vi "testZone.vi"() -> ()   [LabVIEW 2023]
uses:
  zones.ctl
  Zone.lvclass
  Field_class/Field.lvclass
panel:
  out "Zone":T1
  in  "Point":dbl[](array[numeric])
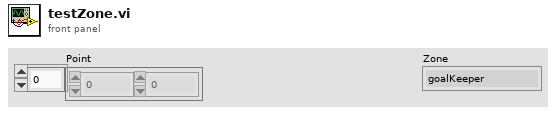
[diagram p1: front panel]
types:
  T1 = typedef "Zone.lvclass/zones.ctl" = enum16{"goalKeeper", "centerBack", "leftBack", "rightBack", "centerMidfield", "leftMidfield", "rightMidfield", "centerForward", "leftWing", "rightWing", "outsideField"}
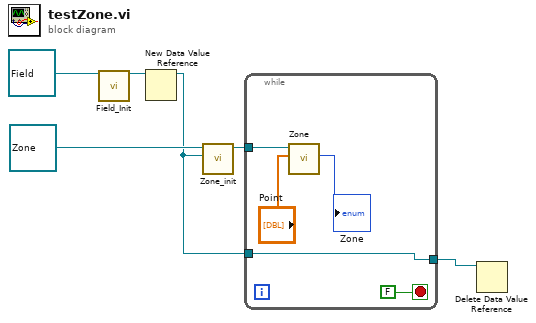
[diagram p0: block diagram]
diagram:
  n1 = call "Field_Init.vi"("object in"=refnum<class "Field.lvclass"> refnum ("Field")) -> ("object out"=w4:refnum<class "Field.lvclass">)  [unwired: 17 in, 1 out]
  n2 = New Data Value Reference(data value=w4) -> (data value reference=w1:refnum<data-value>)  [unwired: 1 in, 1 out]
  n3 = call "Zone_init.vi"("FieldDVR"=w1, "Zone in"=refnum<class "Zone.lvclass"> refnum ("Zone.lvclass")) -> ("Zone out"=w3:refnum<class "Zone.lvclass">)  [unwired: 8 in, 1 out]
  n4 = while {
    tunnel: w3 -> [w10]
    tunnel: [w7] -> w2
    tunnel: w1 -> [w7]
    stop <- FALSE stop-if-true
    n5 = call-dynamic "Zone.vi"("Point"="Point", "Zone in"=w10) -> ("Zone"=→"Zone":T1)  [unwired: 7 in, 2 out]
  }
  n6 = Delete Data Value Reference(data value reference=w2) -> ()  [unwired: 1 in, 2 out]
